vi "Post-Install Custom Action.vi"(10 "Variant":variant) -> (0 "error out":errorcluster)   [LabVIEW 2020]
uses:
  <resource>/dialog/lvconfig.llb/LV Config Write Boolean.vi
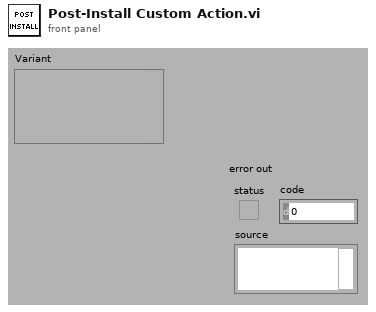
[diagram p1: front panel]
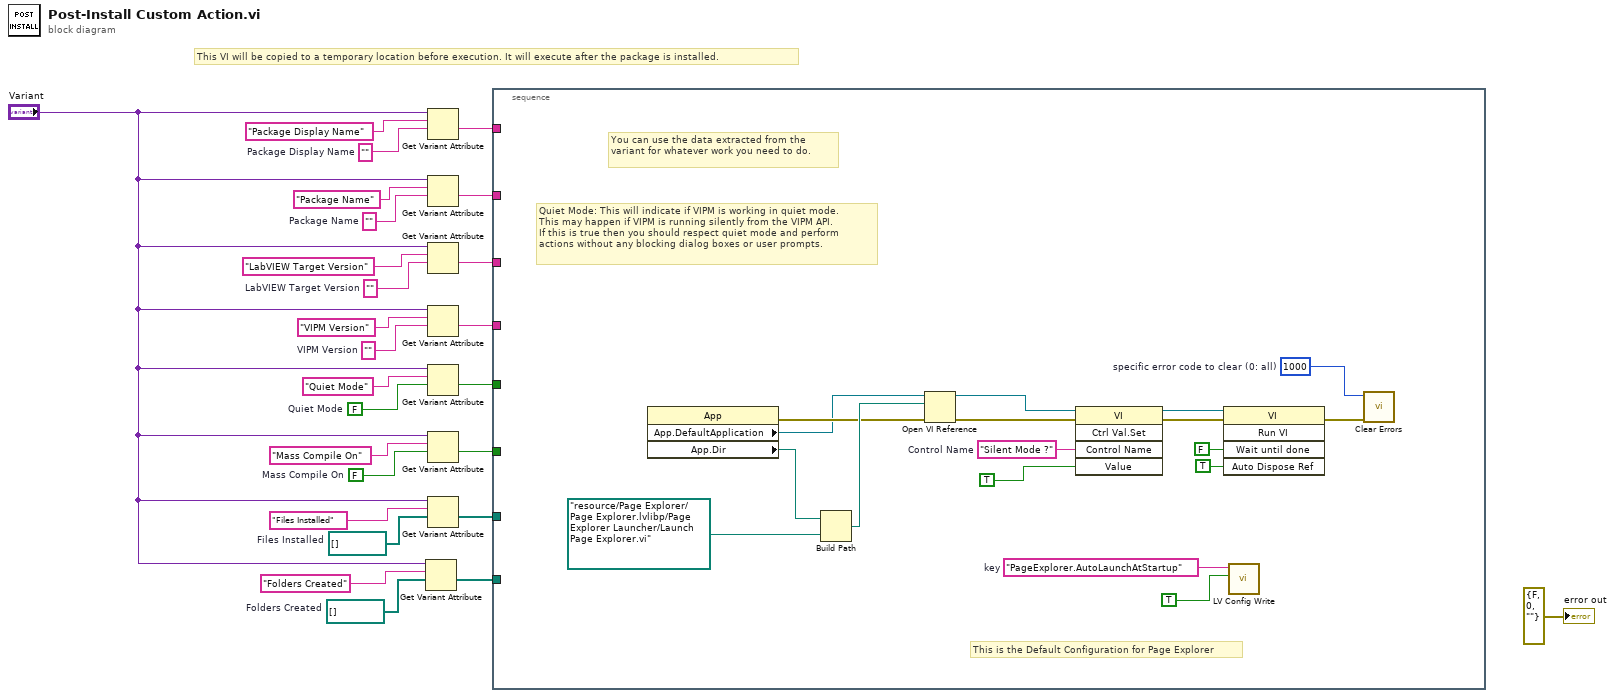
[diagram p0: block diagram]
diagram:
  w1 = path[] []  # Folders Created
  w2 = path[] []  # Files Installed
  w8 = FALSE  # Mass Compile On
  w9 = ""  # Package Display Name
  w16 = FALSE  # Quiet Mode
  w19 = ""  # VIPM Version
  w21 = ""  # LabVIEW Target Version
  w23 = ""  # Package Name
  # "This VI will be copied to a temporary location before execution. It will execute after the package is installed."
  n1 = Get Variant Attribute(Variant="Variant", name="Folders Created", default value (empty Variant)=w1) -> (value=w6:path[])  [unwired: 1 in, 3 out]
  n2 = Get Variant Attribute(Variant="Variant", name="Package Display Name", default value (empty Variant)=w9) -> (value=w15:string)  [unwired: 1 in, 3 out]
  n3 = Get Variant Attribute(Variant="Variant", name="Package Name", default value (empty Variant)=w23) -> (value=w14:string)  [unwired: 1 in, 3 out]
  n4 = Get Variant Attribute(Variant="Variant", name="LabVIEW Target Version", default value (empty Variant)=w21) -> (value=w13:string)  [unwired: 1 in, 3 out]
  n5 = Get Variant Attribute(Variant="Variant", name="VIPM Version", default value (empty Variant)=w19) -> (value=w12:string)  [unwired: 1 in, 3 out]
  n6 = Get Variant Attribute(Variant="Variant", name="Quiet Mode", default value (empty Variant)=w16) -> (value=w11:bool)  [unwired: 1 in, 3 out]
  n7 = Get Variant Attribute(Variant="Variant", name="Mass Compile On", default value (empty Variant)=w8) -> (value=w10:bool)  [unwired: 1 in, 3 out]
  n8 = Get Variant Attribute(Variant="Variant", name="Files Installed", default value (empty Variant)=w2) -> (value=w5:path[])  [unwired: 1 in, 3 out]
  n9 = stacked-sequence {
    tunnel: w15 -> [_]
    tunnel: w14 -> [_]
    tunnel: w13 -> [_]
    tunnel: w12 -> [_]
    tunnel: w11 -> [_]
    tunnel: w10 -> [_]
    tunnel: w5 -> [_]
    tunnel: w6 -> [_]
    frame #0 {
      w29 = 1000  # specific error code to clear (0: all)
      w33 = "Silent Mode ?"  # Control Name
      w43 = "PageExplorer.AutoLaunchAtStartup"  # key
      # "This is the Default Configuration for Page Explorer"
      # "Quiet Mode: This will indicate if VIPM is working in quiet mode.\nThis may happen if VIPM is running silently from the VIPM API.\nIf this is true then you should respect quiet mode and perform\nactions without any blocking dialog boxes or user prompts."
      # "You can use the data extracted from the variant for whatever work you need to do."
      n10 = property class="App"() -> (error out=w38:errorcluster, "App.DefaultApplication"=w28:refnum<vi>, "App.Dir"=w41:path)  [unwired: 2 in, 1 out]
      n11 = Build Path(base path=w41, name or relative path=path "resource/Page Explorer/Page Explorer.lvlibp/Page Explorer Launcher/Launch Page Explorer.vi" ("vi path")) -> (appended path=w39:path)
      n12 = Open VI Reference(application reference (local)=w28, vi path=w39, error in (no error)=w38) -> (vi reference=w31:refnum<vi>, error out=w30:errorcluster)  [unwired: 3 in]
      n13 = invoke class="VI" method="Ctrl Val.Set"(reference=w31, error in=w30, "Control Name"=w33, "Value"=TRUE ("Auto Dispose Reference")) -> (reference out=w34:refnum<vi>, error out=w35:errorcluster)  [unwired: 1 in, 3 out]
      n14 = invoke class="VI" method="Run VI"(reference=w34, error in=w35, "Wait until done"=FALSE ("Wait Until Done"), "Auto Dispose Ref"=TRUE ("Auto Dispose Reference")) -> (error out=w27:errorcluster)  [unwired: 1 in, 4 out]
      n15 = call-poly <resource>:"LV Config Write.vi"("value"=TRUE, "key"=w43) -> ()  [unwired: 5 in, 1 out]
      n16 = call <vilib>:"Clear Errors.vi"("error in (no error)"=w27, "specific error code to clear (0: all)"=w29) -> ()  [unwired: 4 in, 2 out]
    }
  }
  "error out" <- errorcluster {"status"=FALSE, "code"=0, "source"=""} ("error out")
